vi "AppendCallerName.vi"(2 "B":string, 3 "A":string) -> (0 "A.B":string)   [LabVIEW 2025, in "UI_Library.lvlib" / "UI_Library.lvclass"]
doc: "Build Control Name by adding hierarchy caller name\nex:\nA: Cluster\nB: inner boolean\noutput name A.B"
uses:
  UI_Library.lvclass
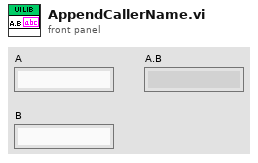
[diagram p1: front panel]
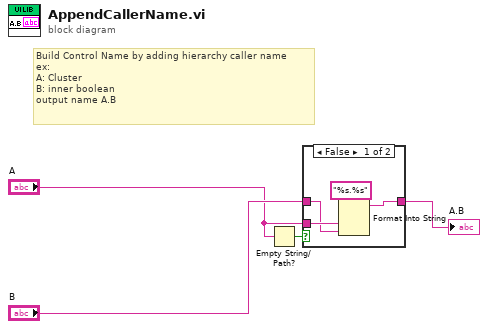
[diagram p0: block diagram]
diagram:
  # "Build Control Name by adding hierarchy caller name\nex:\nA: Cluster\nB: inner boolean\noutput name A.B"
  n1 = Empty String/Path?(string/path="A") -> (empty?=w2:bool)
  n2 = case shown="False" w2 {
    tunnel: "A" -> [w8 _]
    tunnel: "B" -> [w7 w9]
    tunnel: [w5 w9] -> w1
    frame False {
      n3 = Format Into String(format string="%s.%s", w8, w7) -> (resulting string=w5:string)  [unwired: 2 in, 1 out]
    }
    frame True {
    }
  }
  "A.B" <- w1
